vi "RFConfig.vi"(7 "USB-SERIAL name":string="USB-SERIAL", 8 "error in":errorcluster, 10 "接收参数设置":T2, 11 "发射参数设置":T1) -> (0 "error out":errorcluster)   [LabVIEW 2015]
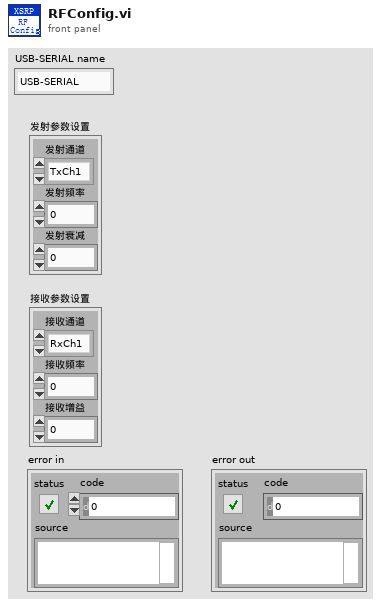
[diagram p1: front panel]
types:
  T1 = cluster{"发射通道":enum16{"TxCh1", "TxCh2"}, "发射频率":u32, "发射衰减":u8}
  T2 = cluster{"接收通道":enum16{"RxCh1", "RxCh2"}, "接收频率":u32, "接收增益":u8}
  T3 = cluster{"端口选择":string, "波特率":u32, "数据位":u16, "奇偶校验":u16, "停止位":u16, "流控":u16}
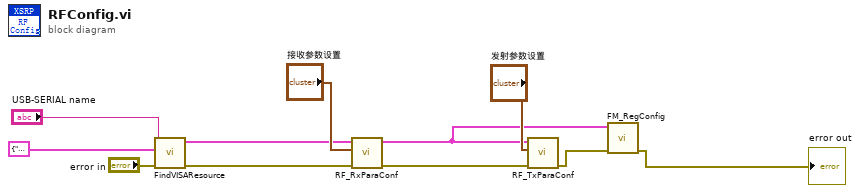
[diagram p0: block diagram]
diagram:
  n1 = call "FindVISAResource.vi"("error in"="error in", "串口配置In"=T3 {"端口选择"="COM2", "波特率"=57600, "数据位"=8, "奇偶校验"=0, "停止位"=10, "流控"=0}, "USB-SERIAL name"="USB-SERIAL name") -> ("error out"=w6:errorcluster, "串口配置Out"=w7:T3)  [unwired: 6 in]
  n2 = call "RF_RxParaConf.vi"("error in"=w6, "DeviceConfiguare"="接收参数设置", "VISA IN"=w7) -> ("error out"=w8:errorcluster, "VISA OUT"=w3:T3)  [unwired: 7 in]
  n3 = call "RF_TxParaConf.vi"("error in"=w8, "硬件\n参数\n设置"="发射参数设置", "VISA IN"=w3) -> ("error OUT"=w1:errorcluster)  [unwired: 8 in]
  n4 = call "FM_RegConfig.vi"("error in"=w1, "VISA IN"=w3) -> ("error out"=→"error out":errorcluster)  [unwired: 8 in, 1 out]
